vi "begin.vi"(7 "field":T1, 9 "lambda":dbl=1e-06, 10 "size_grid":dbl=0.01, 11 "n_grid":i32=256) -> (5 "field out":T1)   [LabVIEW 2012, in "LightPipes.lvlib"]
doc: "__declspec(dllexport) void begin(int n_grid, double size_grid, double lambda, FIELD* field);"
uses:
  LightPipes.lvlib
  <userlib>/LightPipes/LightPipes.dll
panel:
  out "error out":errorcluster
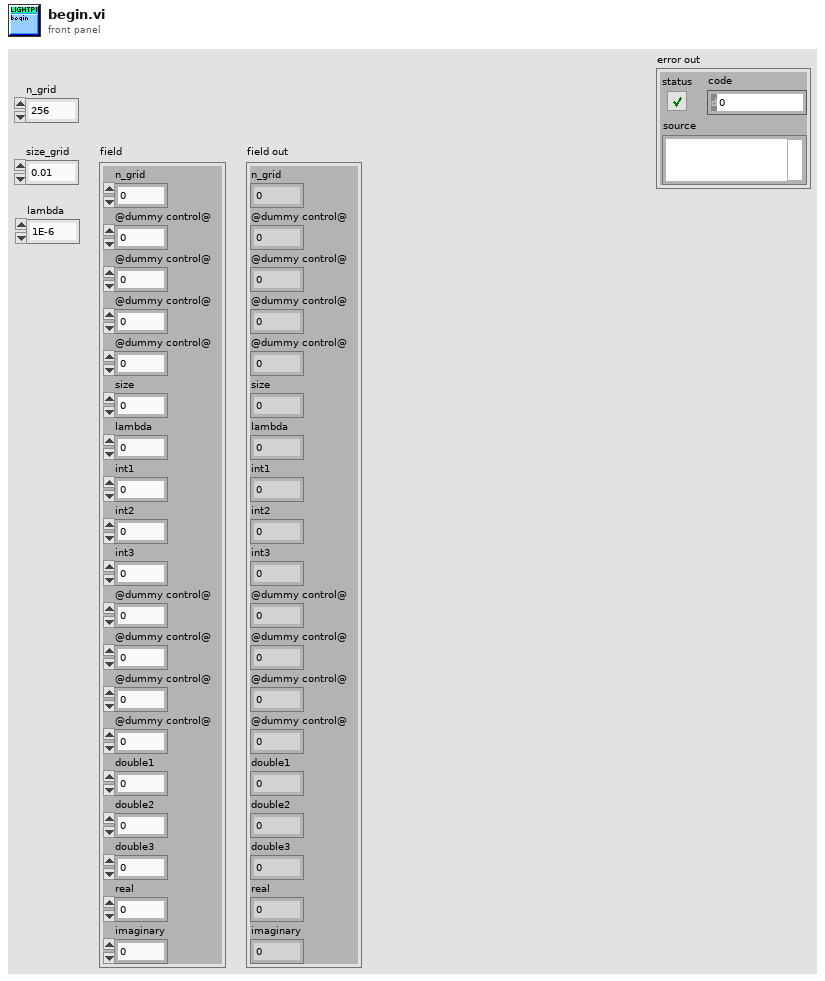
[diagram p1: front panel]
types:
  T1 = cluster{"n_grid":i32, "@dummy control@":i8, "@dummy control@":i8, "@dummy control@":i8, "@dummy control@":i8, "size":dbl, "lambda":dbl, "int1":i32, "int2":i32, "int3":i32, "@dummy control@":i8, "@dummy control@":i8, "@dummy control@":i8, "@dummy control@":i8, "double1":dbl, "double2":dbl, "double3":dbl, "real":u32, "imaginary":u32}
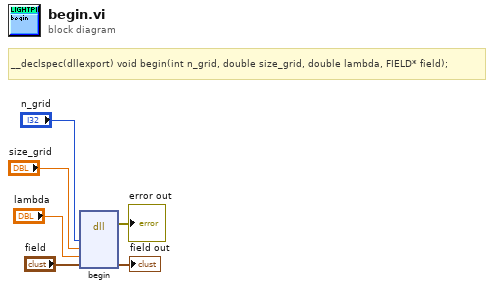
[diagram p0: block diagram]
diagram:
  # "__declspec(dllexport) void begin(int n_grid, double size_grid, double lambda, FIELD* field);"
  n1 = dll-call lib="C:/Program Files (x86)/National Instruments/LabVIEW 2012/user.lib/LightPipes/LightPipes.*" fn="begin"("n_grid"="n_grid", "size_grid"="size_grid", "lambda"="lambda", "field"="field") -> (error out=→"error out":errorcluster, "field"=→"field out":T1)  [unwired: 7 in, 1 out]
